vi "Print Summary.vi"(8 "error in (no error)":errorcluster, 11 "Account in":refnum<class "Account.lvclass">) -> (0 "error out":errorcluster, 2 "Summary":string, 3 "Account out":refnum<class "Account.lvclass">)   [LabVIEW 2017, in "Account.lvclass"]
uses:
  Account.lvclass
  Account.lvclass/Account.ctl
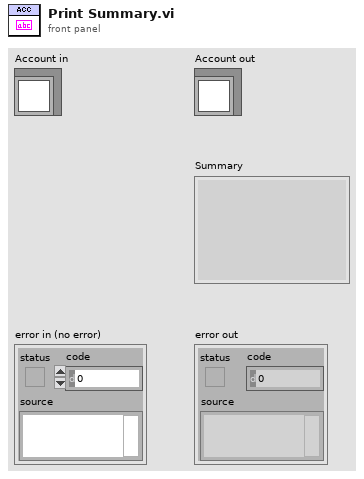
[diagram p1: front panel]
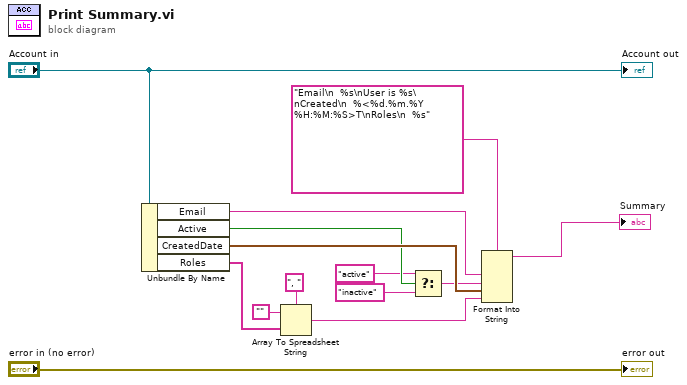
[diagram p0: block diagram]
diagram:
  n1 = Unbundle By Name("Account in") -> ("Email"=w6:string, "Active"=w7:bool, "CreatedDate"=w8:timestamp, "Roles"=w11:string[])
  n2 = Array To Spreadsheet String(delimiter (Tab)=", ", array=w11, 3:"") -> (spreadsheet string=w9:string)
  n3 = Select(t="active", s=w7, f="inactive") -> (s? t:f=w3:string)
  n4 = Format Into String(format string="Email\n  %s\nUser is %s\nCreated\n  %<%d.%m.%Y %H:%M:%S>T\nRoles\n  %s", w6, w3, w8, w9) -> (resulting string=→"Summary":string)  [unwired: 2 in, 1 out]
  "error out" <- "error in (no error)"
  "Account out" <- "Account in"
